vi "Actor Core.vi"(8 "error in":errorcluster, 11 "Instr Actor in":refnum<class "Instr Actor.lvclass">) -> (0 "error out":errorcluster, 3 "Actor out":refnum<class "Actor.lvclass">)   [LabVIEW 2014, in "Instrument.lvlib" / "Instr Actor.lvclass"]
doc: "(<B>Filename</B>: Actor Framework.lvlib:Actor.lvclass:Actor Core.vi)\n\nReceives messages to the actor, reacts to them, and initiates any error handling that may shut the actor down.\n\nDescendant classes may override this VI to append parallel tasks for the actor to complete while it handles messages. Overrides use the Call Parent Method node."
uses:
  Instr Actor.lvclass
  <vilib>/ActorFramework/Actor/Actor.lvclass
  Instr Actor.lvclass/Instr Actor.ctl
  Instrument.lvclass
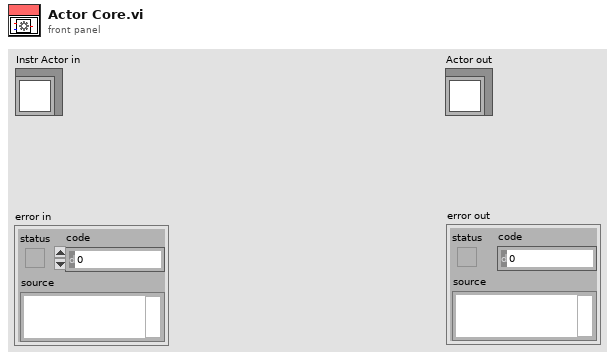
[diagram p1: front panel]
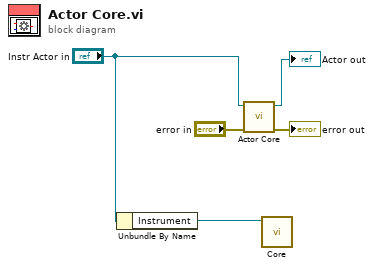
[diagram p0: block diagram]
diagram:
  n1 = Unbundle By Name("Instr Actor in") -> ("Instrument"=w1:refnum<class "Instrument.lvclass">)
  n2 = call-parent "Actor Core.vi"("error in"="error in", "Actor in"="Instr Actor in") -> ("error out"=→"error out":errorcluster, "Actor out"=→"Actor out":refnum<class "Actor.lvclass">)  [unwired: 8 in]
  n3 = call "Core.vi"("Instrument in"=w1) -> ()  [unwired: 11 in]
